vi "Create_Error_log_folders.vi"(3 "Per Day Log File?":bool, 4 "Log Folder":string, 5 "Log Filename":string) -> (0 "exists?":bool, 1 "Server copy Location":path, 2 "Local Log File":path)   [LabVIEW 2010]
uses:
  Globals/Constants_global.vi
  Globals/Preference_global.vi
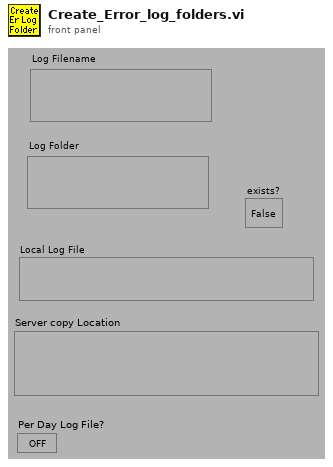
[diagram p1: front panel]
types:
  T1 = cluster{"second":i32, "minute":i32, "hour":i32, "day of month":i32, "month":i32, "year":i32, "day of week":i32, "day of year":i32, "is DST":i32}
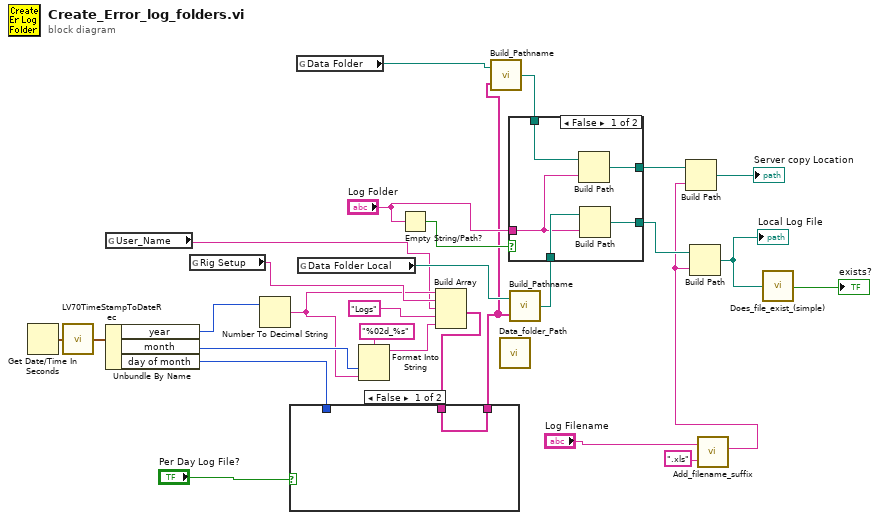
[diagram p0: block diagram]
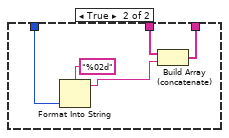
[diagram p2: hidden frame]
diagram:
  n1 = Get Date/Time In Seconds() -> (seconds since 1Jan1904=w2:timestamp)
  n2 = call <vilib>:"LV70TimeStampToDateRec.vi"("time stamp"=w2) -> ("date time rec"=w27:T1)
  n3 = global read "Preference_global.vi" "User_Name"() -> (w1:string)
  n4 = Unbundle By Name(w27) -> ("year"=w26:i32, "month"=w17:i32, "day of month"=w5:i32)
  n5 = global read "Preference_global.vi" "Rig Setup"() -> (w19:string)
  n6 = Number To Decimal String(number=w26) -> (decimal integer string=w16:string)  [unwired: 1 out]
  n7 = global read "Constants_global.vi" "Data Folder"() -> (w11:path)
  n8 = global read "Constants_global.vi" "Data Folder Local"() -> (w25:path)
  n9 = Format Into String(format string="%02d_%s", w17, w16) -> (resulting string=w14:string)  [unwired: 2 in, 1 out]
  n10 = Empty String/Path?(string/path="Log Folder") -> (empty?=w20:bool)
  n11 = Build Array(w16, w19, w1, "Logs", w14) -> (w4:string[])
  n12 = case shown="False" "Per Day Log File?" {
    tunnel: w5 -> [_ w33]
    tunnel: w4 -> [w29 w31]
    tunnel: [w29 w30] -> w3
    frame False {
    }
    frame True {
      n13 = Format Into String(format string="%02d", w33) -> (resulting string=w32:string)  [unwired: 2 in, 1 out]
      n14 = Build Array (concatenate)(w31, w32) -> (w30:string[])
    }
  }
  n15 = call "Build_Pathname.vi"("Output Array"=w3, "Pathname"=w11) -> ("Appended path"=w10:path)
  n16 = call "Data_folder_Path.vi"() -> ()  [unwired: 2 in, 1 out]
  n17 = call "Build_Pathname.vi"("Output Array"=w3, "Pathname"=w25) -> ("Appended path"=w22:path)
  n18 = case shown="False" w20 {
    tunnel: w22 -> [w39 w41]
    tunnel: [w38 w41] -> w28
    tunnel: "Log Folder" -> [w36 _]
    tunnel: w10 -> [w37 w40]
    tunnel: [w35 w40] -> w9
    frame False {
      n19 = Build Path(base path=w37, name or relative path=w36) -> (appended path=w35:path)
      n20 = Build Path(base path=w39, name or relative path=w36) -> (appended path=w38:path)
    }
    frame True {
    }
  }
  n21 = call "Add_filename_suffix.vi"("Filename"="Log Filename", "Suffix to add"=".xls") -> ("Filename out"=w8:string)  [unwired: 3 out]
  n22 = Build Path(base path=w9, name or relative path=w8) -> (appended path=→"Server copy Location":path)
  n23 = Build Path(base path=w28, name or relative path=w8) -> (appended path=w23:path)
  "Local Log File" <- w23
  n24 = call "Does_file_exist_(simple).vi"("Pathname"=w23) -> ("exists?"=→"exists?":bool)
